vi "GatherTrainData.vi"(6 "Function":enum16{"All", "One"}(ring)=enum."One", 9 "uuid":string, 11 "CData Out":T1) -> (1 "Cluster":T2, 2 "Found?":bool, 3 "Array":T3(array[cluster]))   [LabVIEW 2014]
uses:
  DataManager/StateStore/Controls/CData Core Control.ctl
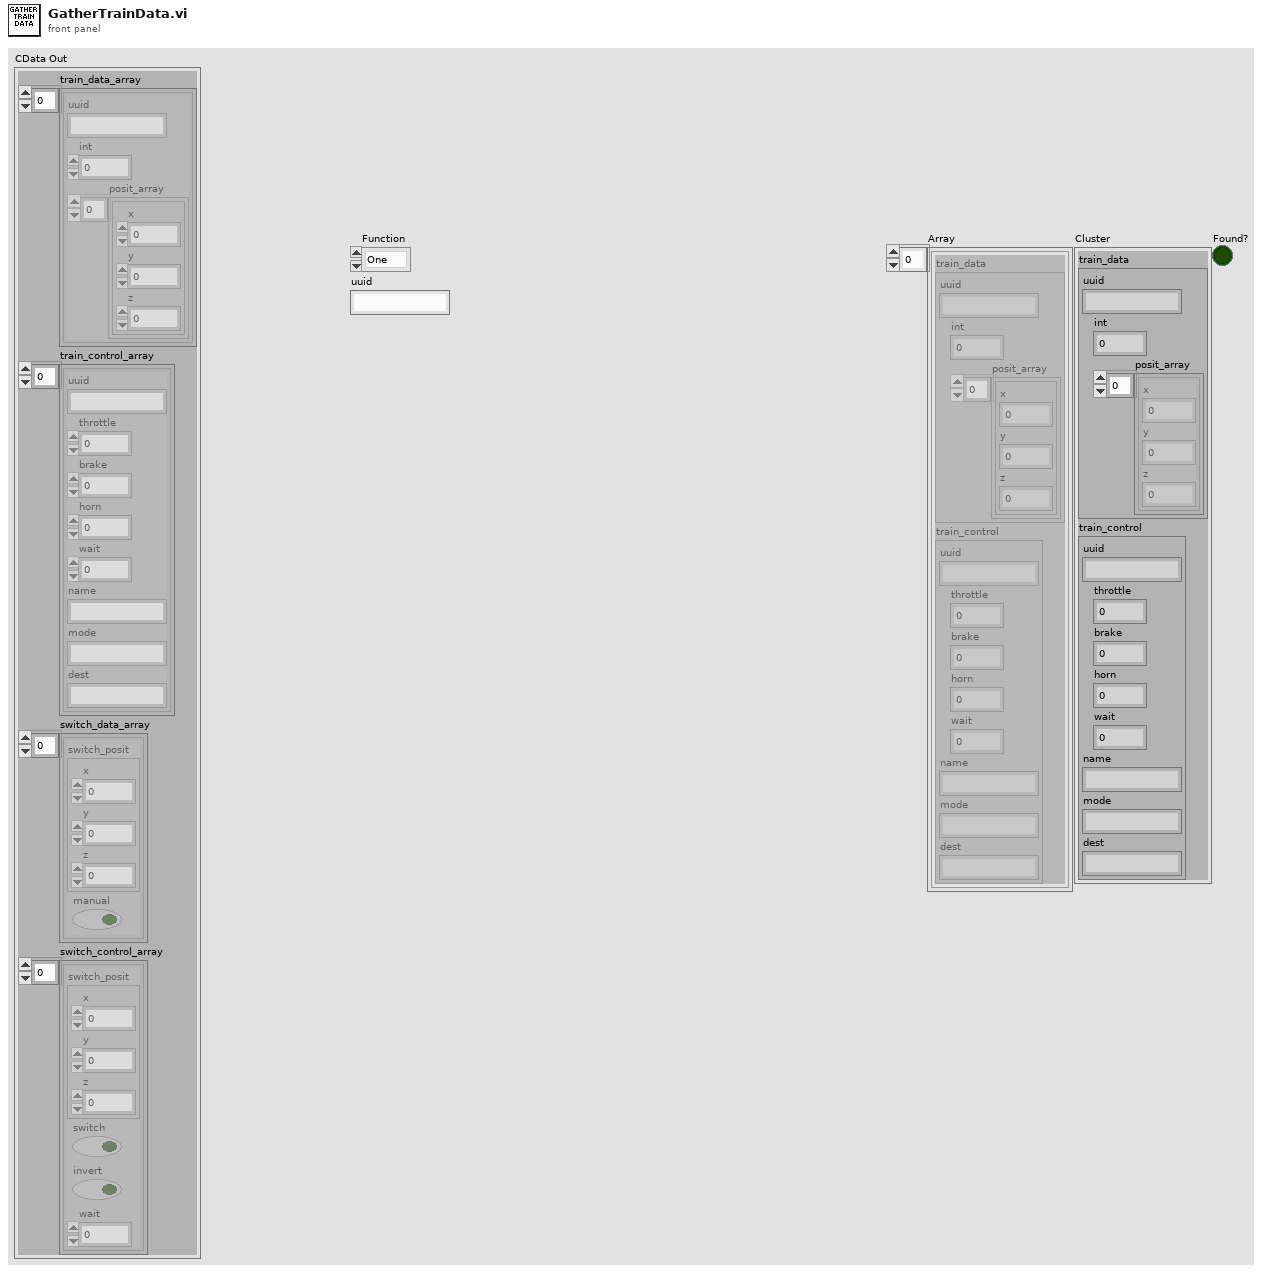
[diagram p1: front panel]
types:
  T1 = typedef "CData Core Control.ctl" = cluster{"train_data_array":cluster{"uuid":string, "int":i32, "posit_array":cluster{"x":dbl, "y":dbl, "z":dbl}[]}[], "train_control_array":cluster{"uuid":string, "throttle":dbl, "brake":dbl, "horn":dbl, "wait":dbl, "name":string, "mode":string, "dest":string}[], "switch_data_array":cluster{"switch_posit":cluster{"x":dbl, "y":dbl, "z":dbl}, "manual":bool}[], "switch_control_array":cluster{"switch_posit":cluster{"x":dbl, "y":dbl, "z":dbl}, "switch":bool, "invert":bool, "wait":dbl}[]}
  T2 = cluster{"train_data":cluster{"uuid":string, "int":i32, "posit_array":cluster{"x":dbl, "y":dbl, "z":dbl}[]}, "train_control":cluster{"uuid":string, "throttle":dbl, "brake":dbl, "horn":dbl, "wait":dbl, "name":string, "mode":string, "dest":string}}
  T3 = cluster{"train_data":cluster{"uuid":string, "int":i32, "posit_array":cluster{"x":dbl, "y":dbl, "z":dbl}[]}, "train_control":cluster{"uuid":string, "throttle":dbl, "brake":dbl, "horn":dbl, "wait":dbl, "name":string, "mode":string, "dest":string}}[]
  T4 = cluster{"uuid":string, "throttle":dbl, "brake":dbl, "horn":dbl, "wait":dbl, "name":string, "mode":string, "dest":string}
  T5 = cluster{"uuid":string, "int":i32, "posit_array":cluster{"x":dbl, "y":dbl, "z":dbl}[]}[]
  T6 = cluster{"uuid":string, "throttle":dbl, "brake":dbl, "horn":dbl, "wait":dbl, "name":string, "mode":string, "dest":string}[]
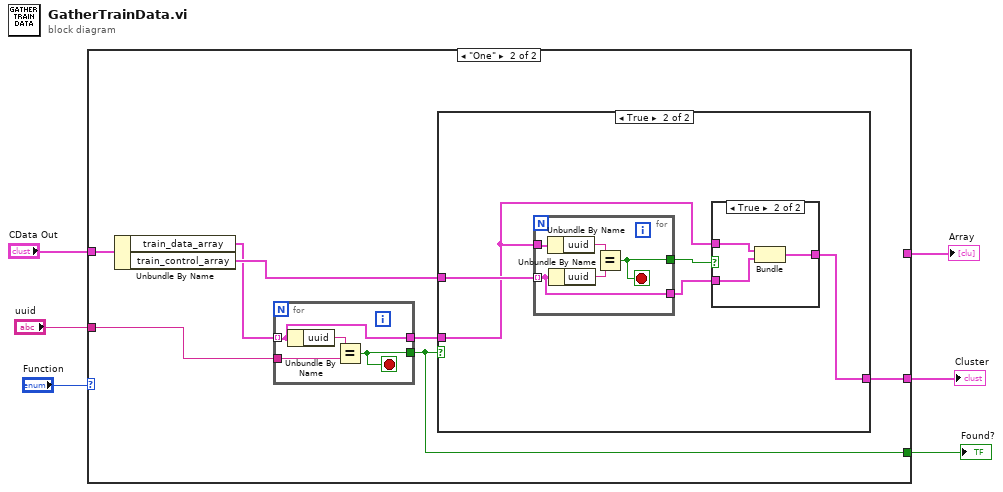
[diagram p0: block diagram]
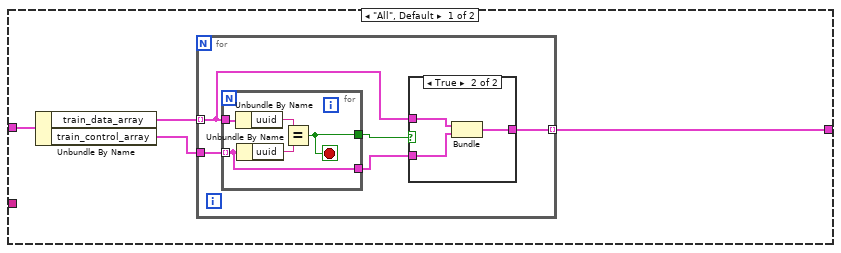
[diagram p2: hidden frame]
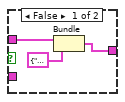
[diagram p3: hidden frame]
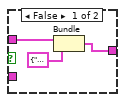
[diagram p5: hidden frame]
diagram:
  n1 = case shown="\"One\"" "Function" {
    tunnel: "CData Out" -> [w8 w32]
    tunnel: [w7 _] -> w6
    tunnel: [_ w27] -> w4
    tunnel: "uuid" -> [_ w30]
    tunnel: [_ w29] -> w2
    frame "All", Default {
      n2 = Unbundle By Name(w8) -> ("train_data_array"=w10:T5, "train_control_array"=w9:T6)
      n3 = for {
        tunnel: w10 -> [w13] mode=indexing
        tunnel: w9 -> [w15]
        tunnel: [w11] -> w7 mode=indexing
        n4 = for {
          tunnel: w13 -> [w26]
          tunnel: w15 -> [w22] mode=indexing
          tunnel: [w23] -> w14
          tunnel: [w22] -> w12
          stop <- w23 stop-if-true
          n5 = Unbundle By Name(w26) -> ("uuid"=w24:string)
          n6 = Unbundle By Name(w22) -> ("uuid"=w25:string)
          n7 = Equal?(x=w24, y=w25) -> (x = y?=w23:bool)
        }
        n8 = case shown="True" w14 {
          tunnel: w13 -> [w18 w21]
          tunnel: w12 -> [_ w20]
          tunnel: [w16 w19] -> w11
          frame False {
            n9 = Bundle("train_data"=w18, "train_control"=T4 {"uuid"="", "throttle"=0.0, "brake"=0.0, "horn"=0.0, "wait"=0.0, "name"="", "mode"="", "dest"=""}) -> (w16:T2)  [unwired: 1 in]
          }
          frame True {
            n10 = Bundle("train_data"=w21, "train_control"=w20) -> (w19:T2)  [unwired: 1 in]
          }
        }
      }
    }
    frame "One" {
      n11 = Unbundle By Name(w32) -> ("train_data_array"=w31:T5, "train_control_array"=w33:T6)
      n12 = for {
        tunnel: w31 -> [w50] mode=indexing
        tunnel: [w52] -> w29
        tunnel: w30 -> [w51]
        tunnel: [w50] -> w28
        stop <- w52 stop-if-true
        n13 = Unbundle By Name(w50) -> ("uuid"=w53:string)
        n14 = Equal?(x=w53, y=w51) -> (x = y?=w52:bool)
      }
      n15 = case shown="True" w29 {
        tunnel: w33 -> [_ w38]
        tunnel: w28 -> [_ w35]
        tunnel: [_ w34] -> w27
        frame False {
        }
        frame True {
          n16 = for {
            tunnel: w35 -> [w49]
            tunnel: w38 -> [w45] mode=indexing
            tunnel: [w46] -> w37
            tunnel: [w45] -> w36
            stop <- w46 stop-if-true
            n17 = Unbundle By Name(w49) -> ("uuid"=w47:string)
            n18 = Unbundle By Name(w45) -> ("uuid"=w48:string)
            n19 = Equal?(x=w47, y=w48) -> (x = y?=w46:bool)
          }
          n20 = case shown="True" w37 {
            tunnel: w35 -> [w41 w44]
            tunnel: w36 -> [_ w43]
            tunnel: [w39 w42] -> w34
            frame False {
              n21 = Bundle("train_data"=w41, "train_control"=T4 {"uuid"="", "throttle"=0.0, "brake"=0.0, "horn"=0.0, "wait"=0.0, "name"="", "mode"="", "dest"=""}) -> (w39:T2)  [unwired: 1 in]
            }
            frame True {
              n22 = Bundle("train_data"=w44, "train_control"=w43) -> (w42:T2)  [unwired: 1 in]
            }
          }
        }
      }
    }
  }
  "Array" <- w6
  "Cluster" <- w4
  "Found?" <- w2
